vi "Is OD Entry.vi"(8 "error in":errorcluster, 11 "Section in":refnum<class "Section.lvclass">) -> (0 "error out":errorcluster, 1 "Is OD Entry?":bool, 2 "Index":u16 format="%.0x", 3 "Section out":refnum<class "Section.lvclass">, 4 "Is Sub-Entry?":bool)   [LabVIEW 2024, in "Electronic Datasheet.lvlib" / "Section.lvclass"]
uses:
  Section.lvclass
  Section.lvclass/Section.ctl
  Section Name/Section Name.lvclass
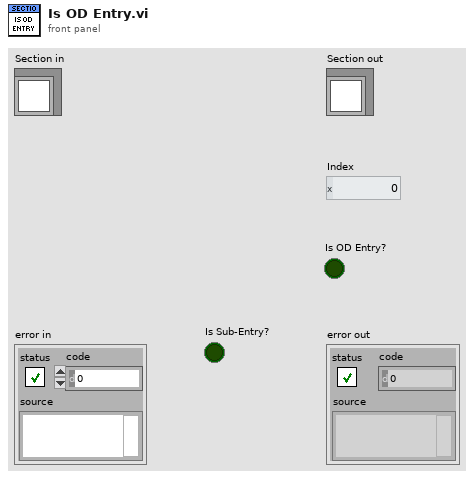
[diagram p1: front panel]
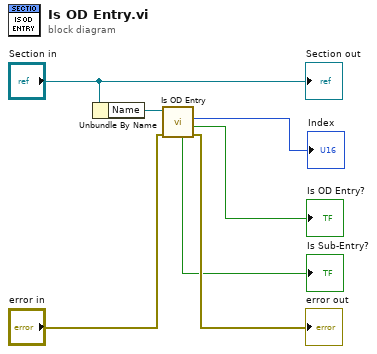
[diagram p0: block diagram]
diagram:
  n1 = Unbundle By Name("Section in") -> ("Name"=w6:refnum<class "Section Name.lvclass">)
  n2 = call "Is OD Entry.vi"("error in"="error in", "Section Name in"=w6) -> ("error out"=→"error out":errorcluster, "Is OD Entry?"=→"Is OD Entry?":bool, "Index"=→"Index":u16, "Is Sub-Entry?"=→"Is Sub-Entry?":bool)  [unwired: 5 in, 1 out]
  "Section out" <- "Section in"
